vi "Agilent Sort Channels.vi"(0 "Agilent Chanel List":string, 5 "Agilent Label List":string[](array[string])) -> (4 "Sorted Channels":string, 6 "Sorted Labels Array":string[](array[string]))   [LabVIEW 2016]
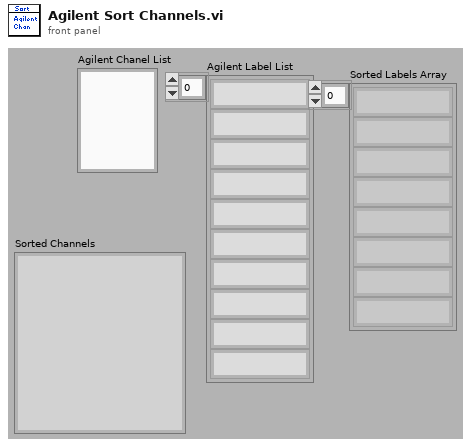
[diagram p1: front panel]
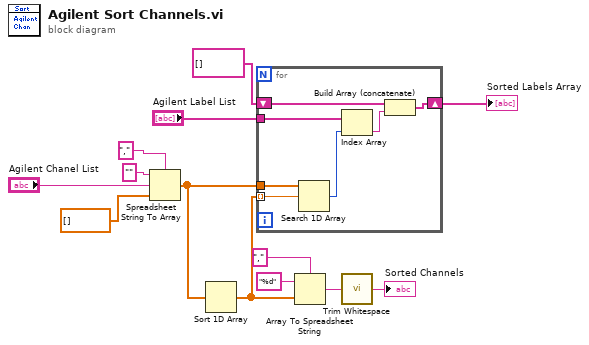
[diagram p0: block diagram]
diagram:
  n1 = Spreadsheet String To Array(delimiter (Tab)=",", format string="", spreadsheet string="Agilent Chanel List", array type (2D Dbl)=dbl[] []) -> (array=w9:dbl[])
  n2 = Sort 1D Array(array=w9) -> (sorted array=w10:dbl[])
  n3 = for {
    tunnel: w10 -> [w19] mode=indexing
    tunnel: w9 -> [w20]
    tunnel: "Agilent Label List" -> [w18]
    shift-right: [w15] -> w6
    shift-left: string[] [] -> [w14]
    n4 = Search 1D Array(1D array=w20, element=w19) -> (index of element=w17:i32)  [unwired: 1 in]
    n5 = Index Array(array=w18, index=w17) -> (element=w16:string)
    n6 = Build Array (concatenate)(w14, w16) -> (w15:string[])
  }
  "Sorted Labels Array" <- w6
  n7 = Array To Spreadsheet String(delimiter (Tab)=",", array=w10, 3:"%d" ("format string")) -> (spreadsheet string=w2:string)
  n8 = call <vilib>:"Trim Whitespace.vi"("string"=w2) -> ("trimmed string"=→"Sorted Channels":string)  [unwired: 1 in]
